vi "Write.ProcessData.vi"(8 "error in":errorcluster, 9 "Offset":i32, 10 "Values":dbl[](array[numeric]), 11 "Write in":refnum<class "Write.lvclass">) -> (0 "error out":errorcluster, 3 "Write out":refnum<class "Write.lvclass">)   [LabVIEW 2027, in "Data Access Engine (Express).lvlib" / "Write.lvclass"]
uses:
  Write.lvclass
  Write.lvclass/Write.ctl
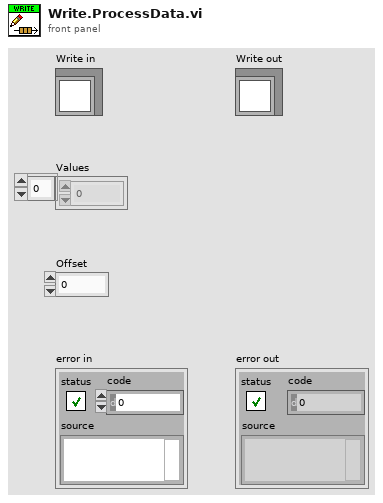
[diagram p1: front panel]
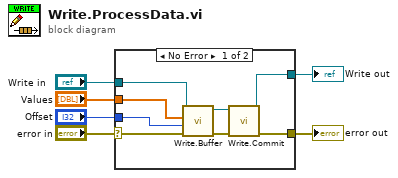
[diagram p0: block diagram]
diagram:
  n1 = case shown="No Error" "error in" {
    selector: "error in" -> [w9 w16]
    tunnel: [w8 w16] -> w5
    tunnel: [w7 w15] -> w3
    tunnel: "Write in" -> [w12 w15]
    tunnel: "Values" -> [w11 _]
    tunnel: "Offset" -> [w10 _]
    frame No Error {
      n2 = call "Write.Buffer.vi"("error in"=w9, "Offset"=w10, "Values"=w11, "Write in"=w12) -> ("error out"=w13:errorcluster, "Write out"=w14:refnum<class "Write.lvclass">)  [unwired: 6 in]
      n3 = call "Write.Commit.vi"("error in"=w13, "Write in"=w14) -> ("error out"=w8:errorcluster, "Write out"=w7:refnum<class "Write.lvclass">)  [unwired: 8 in]
    }
    frame Error {
    }
  }
  "error out" <- w5
  "Write out" <- w3
